vi "getRef.vi"(8 "错误输入（无错误）":errorcluster, 10 "字符串":string, 11 "Gen ref in":refnum<vi>) -> (0 "错误输出":errorcluster, 3 "Gen ref out":refnum<vi>)   [LabVIEW 2017]
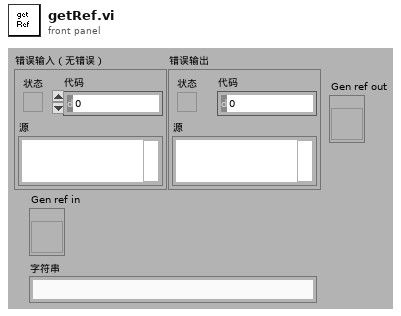
[diagram p1: front panel]
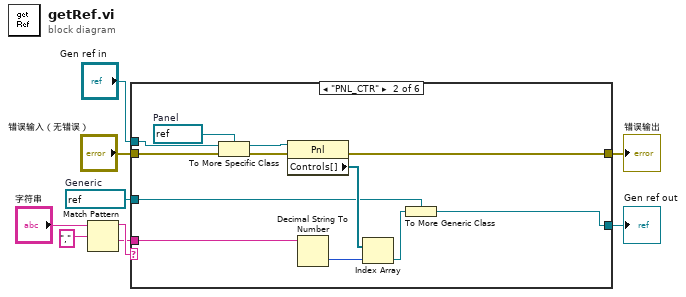
[diagram p0: block diagram]
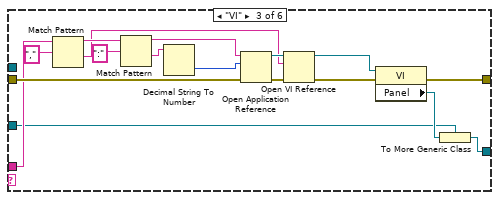
[diagram p3: hidden frame]
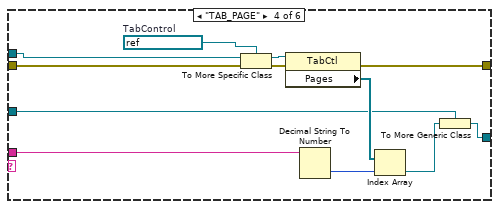
[diagram p4: hidden frame]
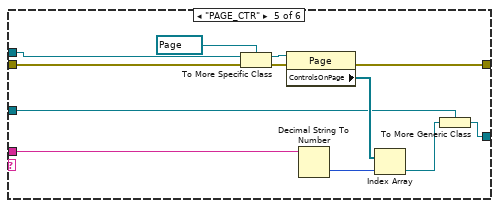
[diagram p5: hidden frame]
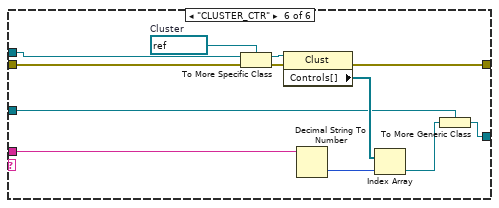
[diagram p6: hidden frame]
diagram:
  w2 = refnum<vi> refnum  # Generic
  n1 = Match Pattern(string="字符串", regular expression="," ("正则表达式")) -> (before substring=w5:string, after substring=w4:string)  [unwired: 3 out]
  n2 = case shown="\"PNL_CTR\"" w5 {
    tunnel: "错误输入（无错误）" -> [w11 w13 w36 w47 w56 w68]
    tunnel: [w11 w16 w25 w42 w54 w67] -> w8
    tunnel: w4 -> [_ w18 w35 w46 w58 w69]
    tunnel: [w10 w22 w28 w44 w60 w66] -> w1
    tunnel: "Gen ref in" -> [w10 w21 _ w48 w62 w72]
    tunnel: w2 -> [_ w15 w24 w41 w53 w70]
    frame "", Default {
    }
    frame "PNL_CTR" {
      w20 = refnum<vi> refnum  # Panel
      n3 = To More Specific Class(target class=w20, reference=w21, error in=w13) -> (specific class reference=w19:refnum<vi>, error out=w12:errorcluster)
      n4 = property class="Pnl"(reference=w19, error in=w12) -> (error out=w16:errorcluster, "Controls[]"=w23:refnum<vi>[])  [unwired: 1 out]
      n5 = Decimal String To Number(string=w18) -> (number=w17:i32)  [unwired: 3 out]
      n6 = Index Array(array=w23, index=w17) -> (element=w14:refnum<vi>)
      n7 = To More Generic Class(target class=w15, reference=w14) -> (generic class reference=w22:refnum<vi>)
    }
    frame "VI" {
      n8 = Match Pattern(string=w35, regular expression="," ("正则表达式")) -> (before substring=w32:string, after substring=w30:string)  [unwired: 3 out]
      n9 = Match Pattern(string=w32, regular expression=":" ("正则表达式")) -> (before substring=w31:string, after substring=w27:string)  [unwired: 3 out]
      n10 = Decimal String To Number(string=w27) -> (number=w26:i32)  [unwired: 3 out]
      n11 = Open Application Reference(8:w36, 10:w26, 11:w31) -> (0:w38:errorcluster, 3:w39:refnum<vi>)  [unwired: 1 out]
      n12 = Open VI Reference(application reference (local)=w39, vi path=w30, error in (no error)=w38) -> (vi reference=w40:refnum<vi>, error out=w37:errorcluster)  [unwired: 3 out]
      n13 = property class="VI"(reference=w40, error in=w37) -> (error out=w25:errorcluster, "Panel"=w29:refnum<vi>)  [unwired: 1 out]
      n14 = To More Generic Class(target class=w24, reference=w29) -> (generic class reference=w28:refnum<vi>)
    }
    frame "TAB_PAGE" {
      w49 = refnum<vi> refnum  # TabControl
      n15 = To More Specific Class(target class=w49, reference=w48, error in=w47) -> (specific class reference=w50:refnum<vi>, error out=w51:errorcluster)
      n16 = property class="TabCtl"(reference=w50, error in=w51) -> (error out=w42:errorcluster, "Pages"=w52:refnum<vi>[])  [unwired: 1 out]
      n17 = Decimal String To Number(string=w46) -> (number=w43:i32)  [unwired: 3 out]
      n18 = Index Array(array=w52, index=w43) -> (element=w45:refnum<vi>)
      n19 = To More Generic Class(target class=w41, reference=w45) -> (generic class reference=w44:refnum<vi>)
    }
    frame "PAGE_CTR" {
      n20 = To More Specific Class(target class=refnum<vi> refnum ("元素"), reference=w62, error in=w56) -> (specific class reference=w61:refnum<vi>, error out=w63:errorcluster)
      n21 = property class="Page"(reference=w61, error in=w63) -> (error out=w54:errorcluster, "ControlsOnPage"=w64:refnum<vi>[])  [unwired: 1 out]
      n22 = Decimal String To Number(string=w58) -> (number=w57:i32)  [unwired: 3 out]
      n23 = Index Array(array=w64, index=w57) -> (element=w59:refnum<vi>)
      n24 = To More Generic Class(target class=w53, reference=w59) -> (generic class reference=w60:refnum<vi>)
    }
    frame "CLUSTER_CTR" {
      w71 = refnum<vi> refnum  # Cluster
      n25 = To More Specific Class(target class=w71, reference=w72, error in=w68) -> (specific class reference=w74:refnum<vi>, error out=w75:errorcluster)
      n26 = property class="Clust"(reference=w74, error in=w75) -> (error out=w67:errorcluster, "Controls[]"=w76:refnum<vi>[])  [unwired: 1 out]
      n27 = Decimal String To Number(string=w69) -> (number=w73:i32)  [unwired: 3 out]
      n28 = Index Array(array=w76, index=w73) -> (element=w65:refnum<vi>)
      n29 = To More Generic Class(target class=w70, reference=w65) -> (generic class reference=w66:refnum<vi>)
    }
  }
  "错误输出" <- w8
  "Gen ref out" <- w1
